vi "Read ADU.vi"(8 "error in (no error)":errorcluster, 11 "MB_Master_TCP in":refnum<class "MB_Master_TCP.lvclass">) -> (0 "error out":errorcluster, 2 "MB_ADU":refnum<class "MB_ADU.lvclass">, 3 "MB_Master_TCP out":refnum<class "MB_Master_TCP.lvclass">)   [LabVIEW 2012, in "MB Master.lvlib" / "MB_Master_TCP.lvclass"]
uses:
  MB_Master_TCP.lvclass
  MB_ADU/MB_ADU.lvclass
  MB_Master_TCP.lvclass/MB_Master_TCP.ctl
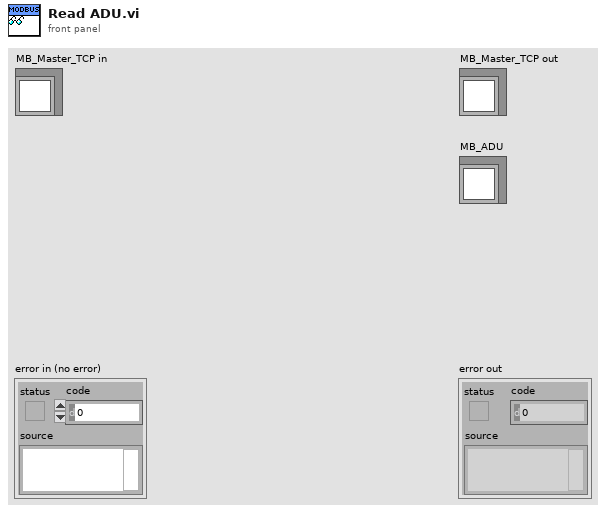
[diagram p1: front panel]
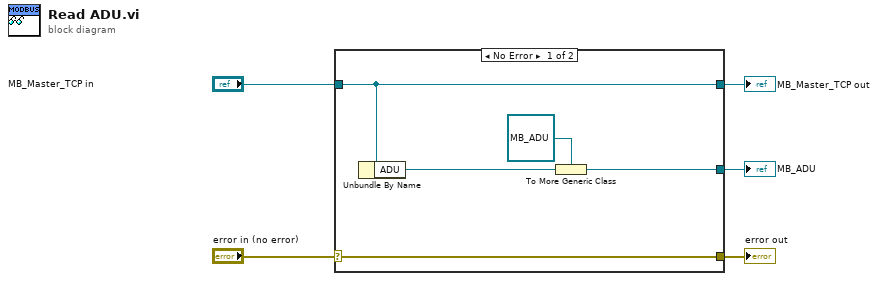
[diagram p0: block diagram]
diagram:
  n1 = case shown="No Error" "error in (no error)" {
    selector: "error in (no error)" -> [w10 w11]
    tunnel: [w10 w11] -> w4
    tunnel: [w9 w12] -> w2
    tunnel: "MB_Master_TCP in" -> [w9 w12]
    tunnel: [w6 _] -> w1
    frame No Error {
      n2 = Unbundle By Name(w9) -> ("ADU"=w8:refnum<class "MB_ADU_TCP.lvclass">)
      n3 = To More Generic Class(target class=refnum<class "MB_ADU.lvclass"> refnum ("MB_ADU"), reference=w8) -> (generic class reference=w6:refnum<class "MB_ADU.lvclass">)
    }
    frame Error {
    }
  }
  "error out" <- w4
  "MB_Master_TCP out" <- w2
  "MB_ADU" <- w1
